vi "Set Center Freq.vi"(8 "error in (no error)":errorcluster, 10 "Center Frequency":u32 format="%#.12p", 11 "RTL-SDR in":refnum<class "Session.lvclass">) -> (0 "error out":errorcluster, 3 "RTL-SDR out":refnum<class "Session.lvclass">)   [LabVIEW 2020, in "RTL-SDR.lvlib" / "Session.lvclass"]
uses:
  Session.lvclass
  C:/dev/IlluminatedG/lv-rtl-sdr/lib/librtlsdr.dll
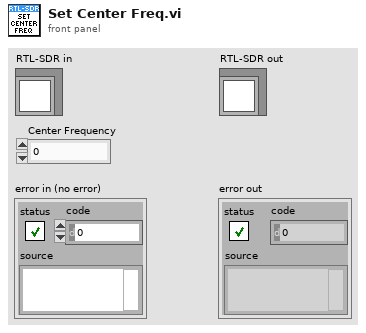
[diagram p1: front panel]
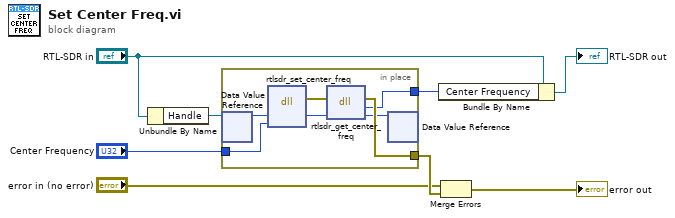
[diagram p0: block diagram]
diagram:
  n1 = Unbundle By Name("RTL-SDR in") -> ("Handle"=w1:refnum<data-value>)
  n2 = in-place {
    in-place-border: [w15] -> w8
    in-place-border: "Center Frequency" -> [w14]
    in-place-border: [w11] -> w3
    n3 = in-place-dvr #1(w1) -> (w10:u64)  [unwired: 1 out]
    n4 = dll-call lib="C:/dev/IlluminatedG/lv-rtl-sdr/lib/librtlsdr.dll" fn="rtlsdr_set_center_freq"("dev"=w10, "freq"=w14) -> (error out=w12:errorcluster, "dev"=w13:u64)  [unwired: 5 in, 1 out]
    n5 = dll-call lib="C:/dev/IlluminatedG/lv-rtl-sdr/lib/librtlsdr.dll" fn="rtlsdr_get_center_freq"(error in=w12, "dev"=w13) -> (error out=w15:errorcluster, "return type"=w11:u32, "dev"=w9:u64)  [unwired: 2 in, 1 out]
    n6 = in-place-dvr #1(w9) -> ()  [unwired: 2 out]
  }
  n7 = Bundle By Name(cluster="RTL-SDR in", "Center Frequency"=w3) -> (→"RTL-SDR out":refnum<class "Session.lvclass">)
  n8 = Merge Errors("error in (no error)", w8) -> (→"error out":errorcluster)
